vi "MD5 File Digest.vi"(8 "error in (no error)":errorcluster, 10 "ChunkSize (10 kB)":i32=10240, 11 "File":path) -> (0 "error out":errorcluster, 2 "MD5 hash":string)   [LabVIEW 2009]
doc: "This VI calculates the MD5 hash of a file"
uses:
  <vilib>/Utility/error.llb/DialogType.ctl
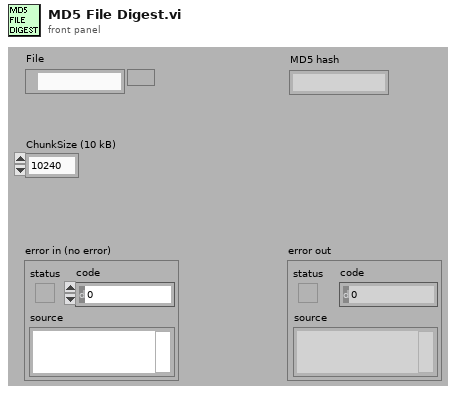
[diagram p1: front panel]
types:
  T1 = typedef "DialogType.ctl" = u16
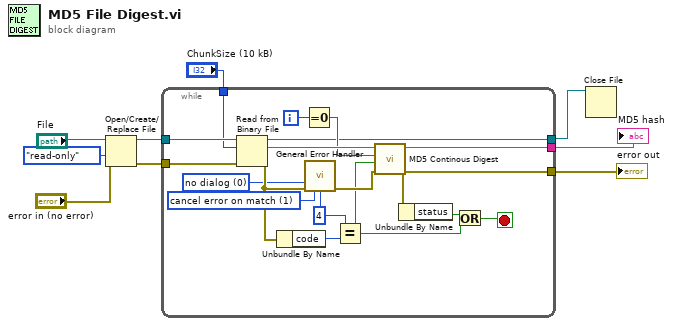
[diagram p0: block diagram]
diagram:
  n1 = Open/Create/Replace File(file path (use dialog)="File", error in="error in (no error)", access (0:read/write)=enum16{"read/write", "read-only", "write-only"}."read-only") -> (refnum out=w8:refnum<file>, error out=w5:errorcluster)  [unwired: 3 in, 1 out]
  n2 = while {
    tunnel: w8 -> [w27]
    tunnel: w5 -> [w26]
    tunnel: "ChunkSize (10 kB)" -> [w25]
    tunnel: [w23] -> w3
    tunnel: [w20] -> w1
    tunnel: [w10] -> w2
    i -> [w22]
    stop <- w11 stop-if-true
    w16 = 1 items=["no exception", "cancel error on match", "set error on match"] ("[exception action] (none:0)")
    w17 = T1 0 items=["no dialog", "OK message", "continue or stop message", "OK message + warnings", "continue/stop + warnings"] ("type of dialog (OK msg:1)")
    w15 = 4 ("y")
    n3 = Read from Binary File(8:w26, 10:w25, 11:w27) -> (0:w18:errorcluster, 2:w24:string, 3:w20:refnum<file>)  [unwired: 3 in, 1 out]
    n4 = Unbundle By Name(w18) -> ("code"=w19:i32)
    n5 = Equal To 0?(x=w22) -> (x = 0?=w21:bool)
    n6 = call <vilib>:"General Error Handler.vi"("type of dialog (OK msg:1)"=w17, "error in (no error)"=w18, "[exception action] (none:0)"=w16, "[exception code]"=w15) -> ("error out"=w14:errorcluster)  [unwired: 7 in, 4 out]
    n7 = Equal?(x=w15, y=w19) -> (x = y?=w12:bool)
    n8 = call "MD5 Continous Digest.vi"("error in (no error)"=w14, "Finish?"=w12, "ReInit?"=w21, "String"=w24) -> ("error out (pass through)"=w10:errorcluster, "MD5 Message Digest"=w23:string)  [unwired: 6 in]
    n9 = Unbundle By Name(w10) -> ("status"=w13:bool)
    n10 = Or(x=w13, y=w12) -> (x .or. y?=w11:bool)
  }
  "error out" <- w2
  "MD5 hash" <- w3
  n11 = Close File(refnum=w1) -> ()  [unwired: 1 in, 2 out]
